vi "Do.vi"(8 "error in (no error)":errorcluster, 10 "Actor in":refnum<class "Actor.lvclass">, 11 "CyclicMessageCountsCycles":refnum<class "MessageCountsExecutions.lvclass">) -> (0 "error out":errorcluster, 2 "Actor out":refnum<class "Actor.lvclass">)   [LabVIEW 2017, in "MessageCountsExecutions.lvclass"]
doc: "(<B>Filename</B>: Actor Framework.lvlib:Message.lvclass:Do.vi)\n\nDefines what a message does when it is received by an actor. Generally, a message instructs an actor to invoke one of its methods. By default, this method does nothing. A child class must override it to define behavior. Create a child class by using the Actor Framework Message Maker dialog box."
uses:
  MessageCountsExecutions.lvclass
  <vilib>/ActorFramework/Actor/Actor.lvclass
  MessageCountsExecutions.lvclass/MessageCountsExecutions.ctl
  <vilib>/ActorFramework/Message/Message.lvclass
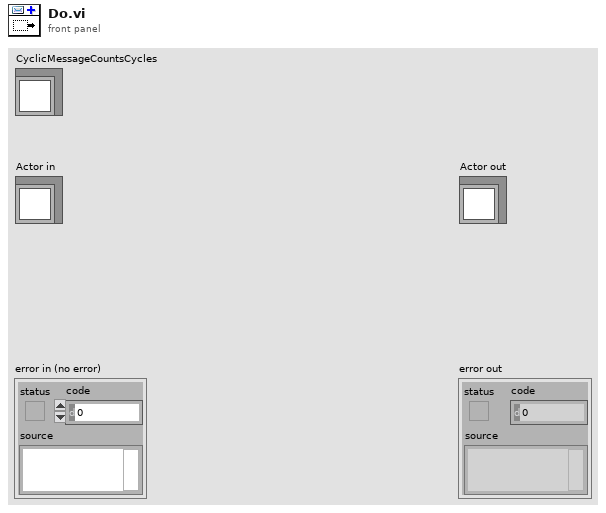
[diagram p1: front panel]
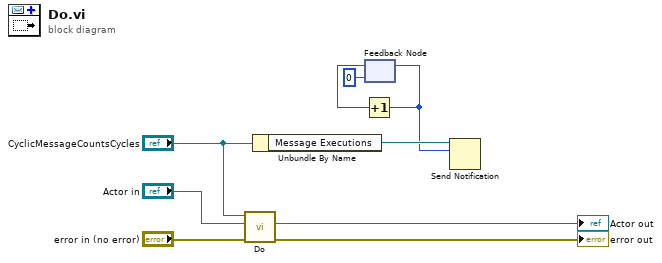
[diagram p0: block diagram]
diagram:
  n1 = call-parent "Do.vi"("error in (no error)"="error in (no error)", "Actor in"="Actor in", "Message"="CyclicMessageCountsCycles") -> ("error out"=→"error out":errorcluster, "Actor out"=→"Actor out":refnum<class "Actor.lvclass">)  [unwired: 7 in]
  n2 = Unbundle By Name("CyclicMessageCountsCycles") -> ("Message Executions"=w4:refnum<notifier>)
  n3 = feedback #1(u32 0) -> (w3:u32)
  n4 = Increment(x=w3) -> (x+1=w1:u32)
  n5 = feedback-in #1(w1) -> ()
  n6 = Send Notification(notification=w1, notifier=w4) -> ()  [unwired: 1 in, 2 out]
